vi "NMVR.vi"(0 "System no.":i32=1 min=1 max=4 step=1, 2 "Axes to move":string[](array[string]), 3 "Position values":dbl[](array[numeric]) format="%.6f", 4 "No.of digits":i16=4, 5 "error in":errorcluster) -> (19 "error out":errorcluster)   [LabVIEW 2020]
doc: "Moves specified axes relative to current position. No. of digits is the number of digits after the decimal point in the position value(s) that will be sent. Uses native move command of controller without any security checks. \n\nE-710: Caution: The use of NMVR.vi is the same as that of the GCS command VI MVR.vi, but it is not a GCS command VI! This function is faster than MVR.vi, but does not check range limits and servo states and does not move the axes synchronously. When the commanded target is outside the range limit, the axis will stop at its physical limit. To go back to normal operation, command the axis to a valid position using MOV.vi. When servo is off, the axis does not move. The commanded target can be queried with MOV?.vi. \nNote: Due to the emulation of the native E-710 command set, the execution of MVR.vi is noticeably slower than that of the native firmware commands. Therefore NMVR.vi is provided for applications which require quickest possible response to motion commands."
panel:
  # "Moves stage relative to actual position. Uses native move \ncommand of controller without any security checks. \nWarning! See VI information for restrictions and risks!"
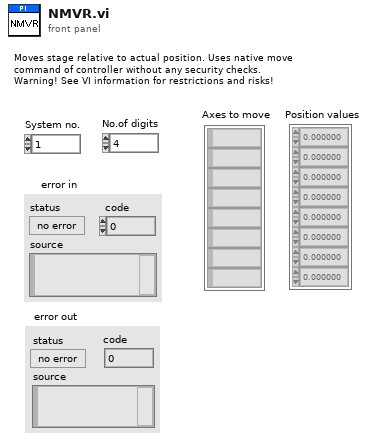
[diagram p1: front panel]
types:
  T1 = enum16{"Disable error check", "Force error check", "Use global settings"}
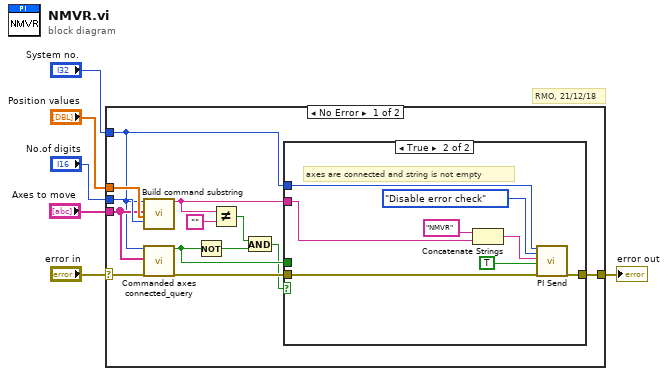
[diagram p0: block diagram]
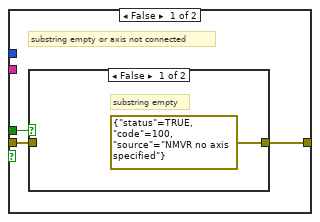
[diagram p2: hidden frame]
diagram:
  # "RMO, 21/12/18"
  n1 = case shown="No Error" "error in" {
    selector: "error in" -> [w7 w33]
    tunnel: [w19 w33] -> w6
    tunnel: "Position values" -> [w16 _]
    tunnel: "No.of digits" -> [w15 _]
    tunnel: "System no." -> [w8 _]
    tunnel: "Axes to move" -> [w13 _]
    frame No Error {
      n2 = call "Build command substring.vi"("System no."=w8, "Affected axes"=w13, "Parameters"=w16, "No. of digits"=w15) -> ("Command substring"=w17:string)  [unwired: 3 in, 12 out]
      n3 = call "Commanded axes connected_query.vi"("System no."=w8, "Commanded axes"=w13, "error in"=w7) -> ("Controller error"=w11:bool, "error out"=w14:errorcluster)  [unwired: 1 in, 14 out]
      n4 = Not(x=w11) -> (.not. x?=w10:bool)
      n5 = Not Equal?(x=w17, y="") -> (x != y?=w12:bool)
      n6 = And(x=w12, y=w10) -> (x .and. y?=w9:bool)
      n7 = case shown="True" w9 {
        tunnel: w17 -> [_ w31]
        tunnel: [w22 w27] -> w19
        tunnel: w14 -> [w20 w28]
        tunnel: w11 -> [w21 _]
        tunnel: w8 -> [_ w26]
        frame False {
          # "substring empty or axis not connected"
          n8 = case shown="False" w21 {
            tunnel: [errorcluster {"status"=TRUE, "code"=100, "source"="NMVR no axis specified"} ("error out") w24] -> w22
            tunnel: w20 -> [_ w24]
            frame False {
              # "substring empty"
            }
            frame True {
              # "commanded axis not connected"
            }
          }
        }
        frame True {
          # "axes are connected and string is not empty"
          n9 = Concatenate Strings("NMVR", w31) -> (w29:string)
          n10 = call "PI Send.vi"("System no."=w26, "Error check settings"=T1."Disable error check", "String to send"=w29, "Attach termination char.?"=TRUE ("Attach Linefeed?"), "error in"=w28) -> ("error out"=w27:errorcluster)  [unwired: 1 in, 13 out]
        }
      }
    }
    frame Error {
    }
  }
  "error out" <- w6
